vi "GetMicronINIPath.vi"(8 "Error In":errorcluster, 11 "Micron Path In":path) -> (0 "Error Out":errorcluster, 2 "Present?":bool, 3 "Micron INI Path Out":path)   [LabVIEW 2019, in "MicronClient.lvclass"]
uses:
  MicronClient.lvclass
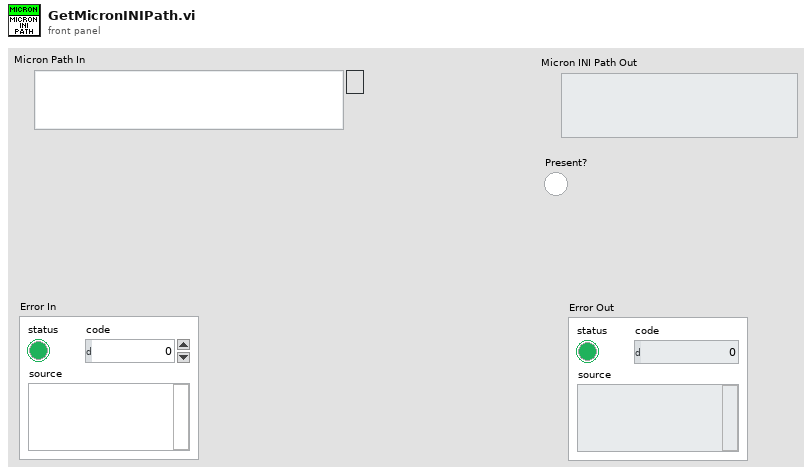
[diagram p1: front panel]
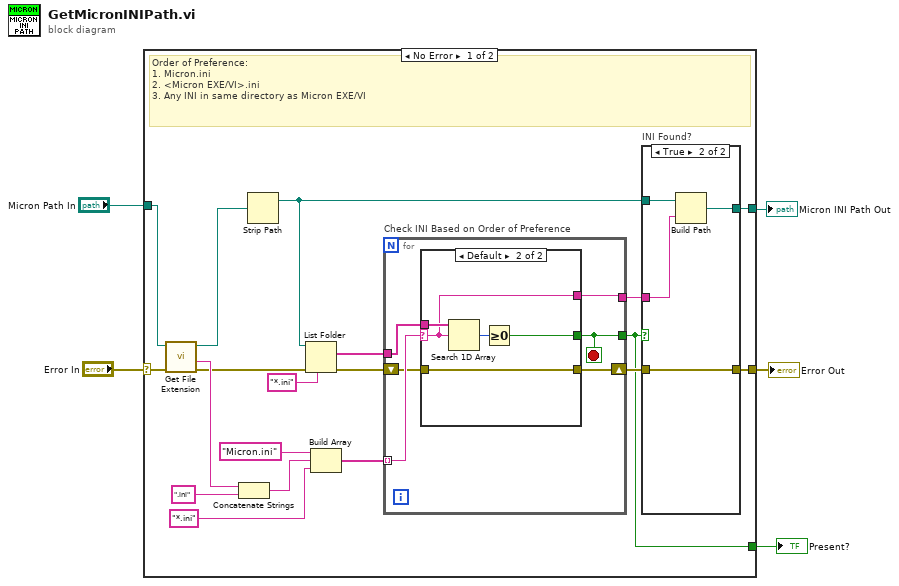
[diagram p0: block diagram]
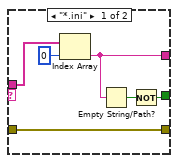
[diagram p3: hidden frame]
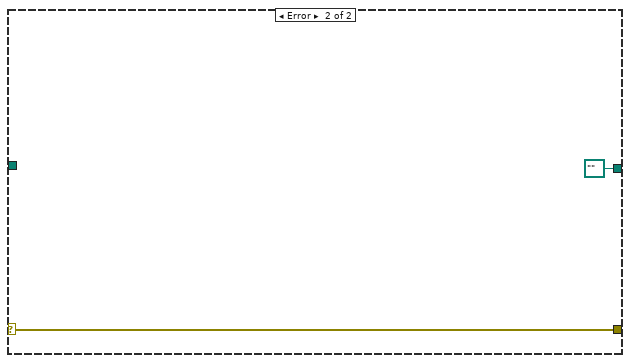
[diagram p4: hidden frame]
diagram:
  n1 = case shown="No Error" "Error In" {
    selector: "Error In" -> [w24 w48]
    tunnel: "Micron Path In" -> [w23 _]
    tunnel: [w7 w48] -> w3
    tunnel: [w8 path "" ("appended path")] -> w2
    tunnel: [w6 _] -> w1
    frame No Error {
      # "Order of Preference:\n1. Micron.ini\n2. <Micron EXE/VI>.ini\n3. Any INI in same directory as Micron EXE/VI"
      n2 = call <vilib>:"Get File Extension.vi"("error in (no error)"=w24, "file"=w23) -> ("error out"=w19:errorcluster, "filename without extension"=w22:string, "dup file"=w20:path)  [unwired: 5 in, 2 out]
      n3 = Concatenate Strings(w22, ".ini" ("string")) -> (w16:string)
      n4 = Strip Path(path=w20) -> (stripped path=w9:path)  [unwired: 1 out]
      n5 = List Folder(path=w9, pattern="*.ini", error in=w19) -> (filenames=w13:string[], error out=w12:errorcluster)  [unwired: 1 in, 2 out]
      n6 = Build Array("Micron.ini", w16, "*.ini") -> (w15:string[])
      n7 = for "Check INI Based on Order of Preference" {
        tunnel: w15 -> [w34] mode=indexing
        tunnel: w13 -> [w35]
        shift-right: [w33] -> w11
        shift-left: w12 -> [w32]
        tunnel: [w31] -> w10
        tunnel: [w30] -> w6
        stop <- w30 stop-if-true
        n8 = case shown="Default" w34 {
          selector: w34 -> [_ w44]
          tunnel: w35 -> [w41 w46]
          tunnel: [w37 w44] -> w31
          tunnel: [w36 w43] -> w30
          tunnel: [w39 w42] -> w33
          tunnel: w32 -> [w39 w42]
          frame "*.ini" {
            n9 = Index Array(array=w41, index=0) -> (element=w37:string)
            n10 = Empty String/Path?(string/path=w37) -> (empty?=w38:bool)
            n11 = Not(x=w38) -> (.not. x?=w36:bool)
          }
          frame Default {
            n12 = Search 1D Array(1D array=w46, element=w44) -> (index of element=w45:i32)  [unwired: 1 in]
            n13 = Greater Or Equal To 0?(x=w45) -> (x >= 0?=w43:bool)
          }
        }
      }
      n14 = case "INI Found?" shown="True" w6 {
        tunnel: w11 -> [w25 w26]
        tunnel: w10 -> [_ w28]
        tunnel: w9 -> [_ w29]
        tunnel: [_ w27] -> w8
        tunnel: [w25 w26] -> w7
        frame False {
        }
        frame True {
          n15 = Build Path(base path=w29, name or relative path=w28) -> (appended path=w27:path)
        }
      }
    }
    frame Error {
    }
  }
  "Error Out" <- w3
  "Micron INI Path Out" <- w2
  "Present?" <- w1
